vi "imtest.vi"() -> ()   [LabVIEW 2018]
panel:
  out "return length":i32
  out "error out":errorcluster
  out "IDN":string
  in  "VISA resource name":refnum<visa-resource-name>
  out "Intensity Graph":u16[][](graph)
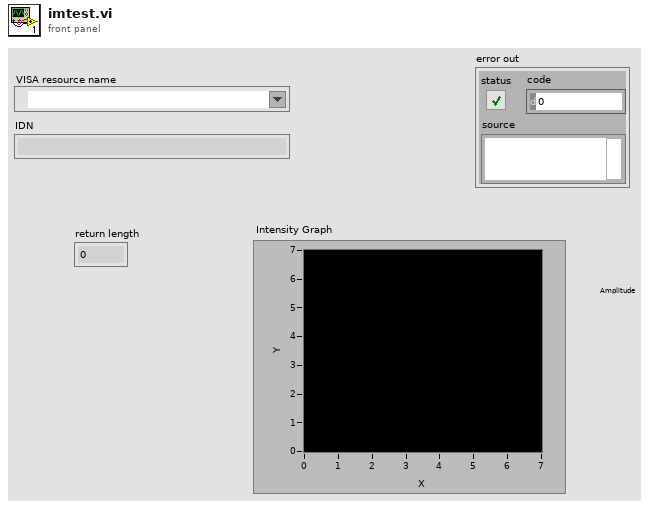
[diagram p1: front panel]
types:
  T1 = enum16{"big-endian, network order", "native, host order", "little-endian"}
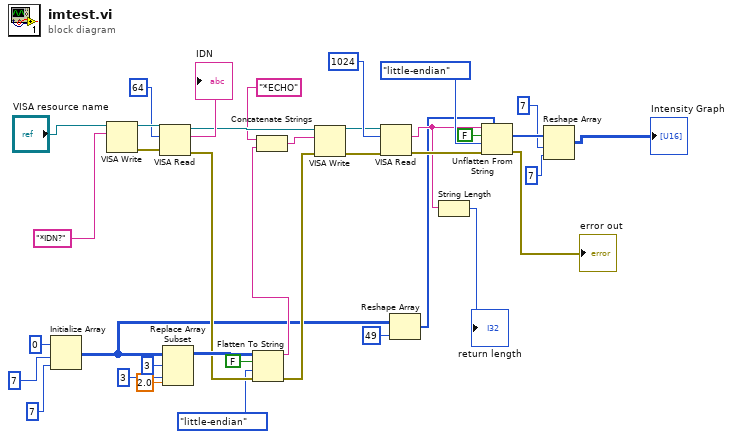
[diagram p0: block diagram]
diagram:
  n1 = Initialize Array(u16 0 ("element"), 7 ("dimension size"), 7 ("dimension size")) -> (w7:u16[][])
  n2 = VISA Write(VISA resource name="VISA resource name", write buffer="*IDN?") -> (VISA resource name out=w32:refnum<visa-resource-name>, error out=w31:errorcluster)  [unwired: 1 in, 1 out]
  n3 = VISA Read(VISA resource name=w32, byte count=64, error in (no error)=w31) -> (VISA resource name out=w21:refnum<visa-resource-name>, read buffer=→"IDN":string, error out=w23:errorcluster)  [unwired: 1 out]
  n4 = Replace Array Subset(array=w7, new element=2.0 ("new element/subarray"), index (row)=3, index (col)=3 ("disabled index (col)")) -> (w25:u16[][])
  n5 = Flatten To String(anything=w25, prepend array or string size? (T)=FALSE, byte order (0:big-endian, network order)=T1."little-endian", error in (no error)=w23) -> (data string=w18:string, error out=w20:errorcluster)  [unwired: 1 out]
  n6 = Concatenate Strings("*ECHO" ("string"), w18) -> (w19:string)
  n7 = VISA Write(VISA resource name=w21, write buffer=w19, error in (no error)=w20) -> (VISA resource name out=w14:refnum<visa-resource-name>, error out=w16:errorcluster)  [unwired: 1 out]
  n8 = VISA Read(VISA resource name=w14, byte count=u32 1024, error in (no error)=w16) -> (read buffer=w9:string, error out=w11:errorcluster)  [unwired: 2 out]
  n9 = Reshape Array(w7, 49 ("dimension size")) -> (w5:u16[])
  n10 = String Length(string=w9) -> (length=→"return length":i32)
  n11 = Unflatten From String(type=w5, binary string=w9, data includes array or string size? (T)=FALSE, byte order (0:big-endian, network order)=T1."little-endian", error in (no error)=w11) -> (value=w4:u16[], error out=→"error out":errorcluster)  [unwired: 1 out]
  n12 = Reshape Array(w4, 7 ("dimension size"), 7 ("dimension size")) -> (→"Intensity Graph":u16[][])
